vi "Quad Ctr, Index Save (subVI).vi"(2 "Reset":bool, 3 "Input Z":bool, 4 "Input B":bool, 5 "Input A":bool) -> (0 "Index Save":i16, 1 "16 bit Position":i16)   [LabVIEW 2015]
doc: "This subVI supports a quadrature decoder application with an indexed save feature. On every valid index state (defined when Input A, Input B and Input Z are all low), the 16 bit Position is saved in the Index Save. The Reset control resets the position asynchronously."
panel:
  # "This subVI supports a quadrature decoder application with an indexed save feature.  On every valid index state (defined when Input A, Input B and Input Z are all low), the 16 bit Position is saved in the Index Save.  The Reset control resets the position asynchronously."
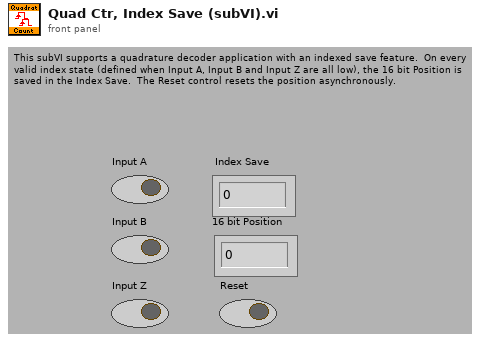
[diagram p1: front panel]
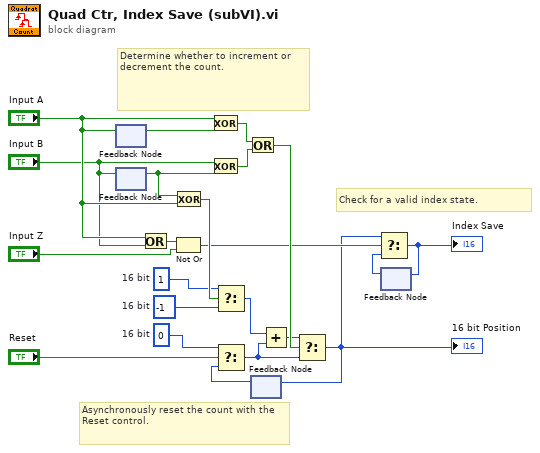
[diagram p0: block diagram]
diagram:
  w16 = i16 -1  # 16 bit
  w15 = i16 1  # 16 bit
  w11 = i16 0  # 16 bit
  # "Asynchronously reset the count with the Reset control."
  # "Check for a valid index state."
  # "Determine whether to increment or decrement the count."
  n1 = feedback-in #1("Input A") -> ()
  n2 = feedback #1() -> (w9:bool)  [unwired: 1 out]
  n3 = feedback-in #2("Input B") -> ()
  n4 = feedback #2() -> (w5:bool)  [unwired: 1 out]
  n5 = Or(x="Input A", y="Input B") -> (x .or. y?=w21:bool)
  n6 = Not Or(1:"Input Z", 2:w21) -> (0:w4:bool)
  n7 = Exclusive Or(1:"Input A", 2:w5) -> (0:w20:bool)
  n8 = Exclusive Or(1:w9, 2:"Input A") -> (0:w18:bool)
  n9 = Exclusive Or(1:w5, 2:"Input B") -> (0:w17:bool)
  n10 = Select(t=w15, s=w20, f=w16) -> (s? t:f=w14:i16)
  n11 = Or(x=w18, y=w17) -> (x .or. y?=w19:bool)
  n12 = feedback #3() -> (w7:i16)  [unwired: 1 out]
  n13 = Select(t=w11, s="Reset", f=w7) -> (s? t:f=w12:i16)
  n14 = Add(x=w14, y=w12) -> (x+y=w10:i16)
  n15 = Select(t=w10, s=w19, f=w12) -> (s? t:f=w2:i16)
  "16 bit Position" <- w2
  n16 = feedback-in #3(w2) -> ()
  n17 = feedback #4() -> (w3:i16)  [unwired: 1 out]
  n18 = Select(t=w2, s=w4, f=w3) -> (s? t:f=w1:i16)
  "Index Save" <- w1
  n19 = feedback-in #4(w1) -> ()
